vi "Generate_SN.vi"(8 "error in (no error)":errorcluster caption="entrée d'erreur (pas d'erreur)", 11 "Class Creation_SN (Default) en entrée":refnum<class "Creation_SN_P2265.lvclass">) -> (0 "error out":errorcluster caption="sortie d'erreur", 3 "Class Creation_SN (Default) en sortie":refnum<class "Creation_SN_P2265.lvclass">)   [LabVIEW 2020, in "Library Instrument & Equipement.lvlib" / "Library Creation_SN.lvlib" / "Creation_SN_P2265.lvclass"]
uses:
  Creation_SN_P2265.lvclass
  C:/Users/ngarcin/OneDrive - Altyor/Standard TB/Class/Creation_SN/Creation_SN Database (Default)/Creation_SN Database (Default).lvclass
  C:/Users/ngarcin/OneDrive - Altyor/Standard TB/Class/Creation_SN/Creation_SN (Default)/Creation_SN (Virtual).lvclass
  Creation_SN Database (Default)/Creation_SN Database (Default).lvclass
  Firebase/Source/Firebase Recovery_SN/Firebase Recovery_SN.lvclass
  Creation_SN_P2265.lvclass/Creation_SN_P2265.ctl
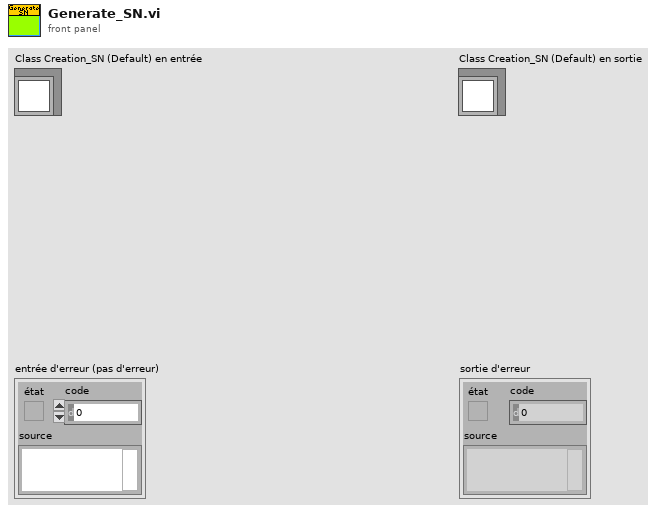
[diagram p1: front panel]
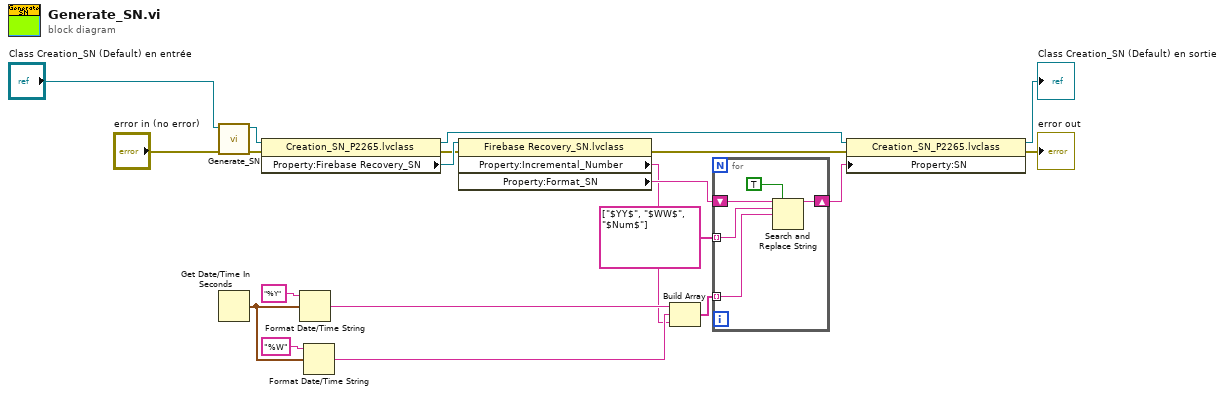
[diagram p0: block diagram]
diagram:
  n1 = call-parent "Generate_SN.vi"("error in (no error)"="error in (no error)", "Class Creation_SN (Default) en entrée"="Class Creation_SN (Default) en entrée") -> ("error out"=w7:errorcluster, "Class Creation_SN (Default) en sortie"=w9:refnum<class "Creation_SN_P2265.lvclass">)  [unwired: 8 in]
  n2 = Get Date/Time In Seconds() -> (seconds since 1Jan1904=w16:timestamp)
  n3 = property class="Creation_SN_P2265.lvclass"(reference=w9, error in=w7) -> (reference out=w5:refnum<class "Creation_SN_P2265.lvclass">, error out=w6:errorcluster, "Property:Firebase Recovery_SN"=w8:refnum<class "Firebase Recovery_SN.lvclass">)
  n4 = Format Date/Time String(time format string (%c)="%Y" ("chaîne de format de l'heure (%c)"), seconds (now)=w16) -> (date/time string=w15:string)  [unwired: 1 in]
  n5 = Format Date/Time String(time format string (%c)="%W" ("chaîne de format de l'heure (%c)"), seconds (now)=w16) -> (date/time string=w14:string)  [unwired: 1 in]
  n6 = property class="Firebase Recovery_SN.lvclass"(reference=w8, error in=w6) -> (error out=w4:errorcluster, "Property:Incremental_Number"=w10:string, "Property:Format_SN"=w11:string)  [unwired: 1 out]
  n7 = Build Array(w15, w14, w10) -> (w13:string[])
  n8 = for {
    tunnel: w13 -> [w24] mode=indexing
    tunnel: string[] ["$YY$", "$WW$", "$Num$"] -> [w25] mode=indexing
    shift-right: [w22] -> w2
    shift-left: w11 -> [w23]
    n9 = Search and Replace String(replace all?=TRUE ("tout remplacer ? (F)"), input string=w23, search string=w25, replace string=w24) -> (result string=w22:string)  [unwired: 4 in, 3 out]
  }
  n10 = property class="Creation_SN_P2265.lvclass"(reference=w5, error in=w4, "Property:SN"=w2) -> (reference out=→"Class Creation_SN (Default) en sortie":refnum<class "Creation_SN_P2265.lvclass">, error out=→"error out":errorcluster)
